vi "pf_Close.vi"(8 "error in (no error)":errorcluster, 11 "IMAQ Session in":refnum<k11>) -> (0 "error out":errorcluster)   [LabVIEW 2025, in "Photonfocus_Toolkit.lvlib"]
doc: "Closes the communication with the camera."
uses:
  Photonfocus_Toolkit.lvlib
  _Private/Controls/pf_Camera_ctrl_mngr_action.ctl
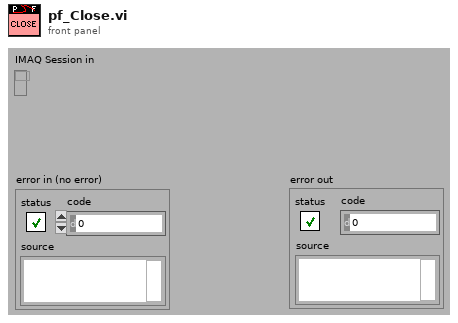
[diagram p1: front panel]
types:
  T1 = typedef "Photonfocus_Toolkit.lvlib/pf_Camera_ctrl_mngr_action.ctl" = enum16{"Create", "Destroy", "Set", "Get"}
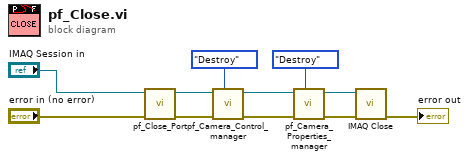
[diagram p0: block diagram]
diagram:
  n1 = call "pf_Close_Port.vi"("error in (no error)"="error in (no error)", "IMAQ Session in"="IMAQ Session in") -> ("error out"=w6:errorcluster, "IMAQ Session out"=w4:refnum<k11>)  [unwired: 8 out]
  n2 = call "pf_Camera_Control_manager.vi"("Action"=pf_Camera_ctrl_mngr_action."Destroy", "error in (no error)"=w6, "IMAQ Session in"=w4) -> ("error out"=w8:errorcluster, "IMAQ Session out"=w9:refnum<k11>)  [unwired: 1 in, 6 out]
  n3 = call "pf_Camera_Properties_manager.vi"("Action"=pf_Camera_ctrl_mngr_action."Destroy", "error in (no error)"=w8, "IMAQ Session in"=w9) -> ("error out"=w2:errorcluster, "IMAQ Session out"=w3:refnum<k11>)  [unwired: 2 in, 5 out]
  n4 = call <vilib>:"IMAQ Close.vi"("error in (no error)"=w2, "IMAQ Session In"=w3) -> ("error out"=→"error out":errorcluster)  [unwired: 9 out]
